vi "m2Triangle.vi"() -> ()   [LabVIEW 2015]
uses:
  Common_RT_ILC/DataTypes/ILCTelemetry.ctl
  Common_RT_ILC/DataTypes/ILCResponses.ctl
  Common_RT_Modbus/DataTypes/ExceptionCodes.ctl
  Common_RT_HPILC/DataTypes/HPResponses.ctl
  Common_RT_HPILC/DataTypes/HPTelemetry.ctl
  Common_RT_HealthAndStatus/RTHealthAndStatus/RTHealthAndStatus.lvclass
  MyHealthAndStatusReadFIFO/MyHealthAndStatusReadFIFO.lvclass
  MyHealthAndStatusWriteFIFO/MyHealthAndStatusWriteFIFO.lvclass
  Common_RT_Modbus/Modbus/Modbus.lvclass
  ModbusPort1ReadFIFO/ModbusPort1ReadFIFO.lvclass
  ModbusPort1WriteFIFO/ModbusPort1WriteFIFO.lvclass
  SoftwareControlledTrigger/SoftwareControlledTrigger.lvclass
  Common_RT_HPILC/HPILCFactory/HPILCFactory.lvclass
  Common_RT_HPILC/DataTypes/HPSettings.ctl
  Common_RT_ILC/DataTypes/ILCSettings.ctl
  SoftwareControlledTrigger/SoftwareControlledTrigger.lvclass/SoftwareControlledTrigger.ctl
  ModbusPort1WriteFIFO/ModbusPort1WriteFIFO.lvclass/ModbusPort1WriteFIFO.ctl
  ModbusPort1ReadFIFO/ModbusPort1ReadFIFO.lvclass/ModbusPort1ReadFIFO.ctl
  MyHealthAndStatusWriteFIFO/MyHealthAndStatusWriteFIFO.lvclass/MyHealthAndStatusWriteFIFO.ctl
  MyHealthAndStatusReadFIFO/MyHealthAndStatusReadFIFO.lvclass/MyHealthAndStatusReadFIFO.ctl
  Common_RT_HealthAndStatus/RTHealthAndStatus/RTHealthAndStatus.lvclass/RTHealthAndStatus.ctl
  Common_RT_ILC/ILC/ILC.lvclass/ILC.ctl
  Common_RT_Modbus/DynamicFrameParser/DynamicFrameParser.lvclass
  Common_RT_HPILC/HPILC/HPILC.lvclass/HPILC.ctl
  <vilib>/FPGAPlugInAG/cRIO-9038/niLvFpga_Open_cRIO-9038.vi
  <vilib>/rvi/interface/common/dynamic/niFpgaDynamicAddResources.vi
  <vilib>/FPGAPlugInAG/Dynamic/niLvFpga_Abort_Dynamic.vi
  <vilib>/FPGAPlugInAG/Dynamic/niLvFpga_Reset_Dynamic.vi
  <vilib>/FPGAPlugInAG/Dynamic/niLvFpga_Run_Dynamic.vi
  <vilib>/Utility/error.llb/Error Cluster From Error Code.vi
  <vilib>/RVI Host/nirviSupport.llb/nirviErrorClusterFromErrorCode.vi
  <vilib>/rvi/errors/niLvFpgaAdjustHostInterfaceError.vi
  <vilib>/FPGAPlugInAG/Dynamic/niLvFpga_Close_Dynamic.vi
  <vilib>/rvi/interface/nirviOpenFPGA/nirviOpenFPGA.xnode
  FPGA Bitfiles/Modbus-4Port.lvbitx
  FPGA/main.vi
  <vilib>/rvi/interface/nirviMethod/nirviMethod.xnode
  <vilib>/rvi/interface/nirviCloseFPGA/nirviCloseFPGA.xnode
  Common_RT_HPILC/HPILC/HPILC.lvclass
  Common_RT_ILC/RTILC.lvlib
  <vilib>/rvi/interface/nirviMethod/StockFPGA_InlinedMethodWaitForSingleIRQ.vi
  <vilib>/FPGAPlugInAG/Dynamic/niLvFpga_WaitOnIrq_Dynamic.vi
  <vilib>/FPGAPlugInAG/Dynamic/niLvFpga_AcknowledgeIrq_Dynamic.vi
  Common_RT_ILC/ILC/ILC.lvclass
  Common_RT_HPILC/RTHPILC.lvlib
  Common_RT_Modbus/RTModbus.lvlib
panel:
  out "minMinEncoder":i32
  out "maxMinEncoder":i32
  out "minMaxEncoder":i32
  out "maxMaxEncoder":i32
  out "Exception on Force and Status":bool
  out "minAvgDelta":dbl
  out "maxAvgDelta":dbl
  out "minMaxDelta":i32
  out "maxMaxDelta":i32
  out "minMinDelta":i32
  out "maxMinDelta":i32
  out "MaxDelta":i32(graph)
  out "MinDelta":i32(graph)
  out "AvgDelta":dbl(graph)
  out "avgDelta":dbl
  out "minDelta":i32
  out "maxDelta":i32
  out "minValue":i32
  out "maxValue":i32
  out "Encoder":i32(graph)
  out "Steps":i32
  in  "Stop":bool
  out "HPTelemetry":T1
  out "HPResponses":T2
  in  "Boolean":bool
  out "ILCResponses":T4
  out "ILCTelemetry":T5
  out "Port 1 Status Bits":u64 format="%016b"
  out "error out":errorcluster
  out "Port 1 Frames Received":i64
  out "Port 1 Bytes Received":i64
  out "Port 1 Frames Transmitted":i64
  out "Port 1 Bytes Transmitted":i64
  # "Port 1 = Modbus"
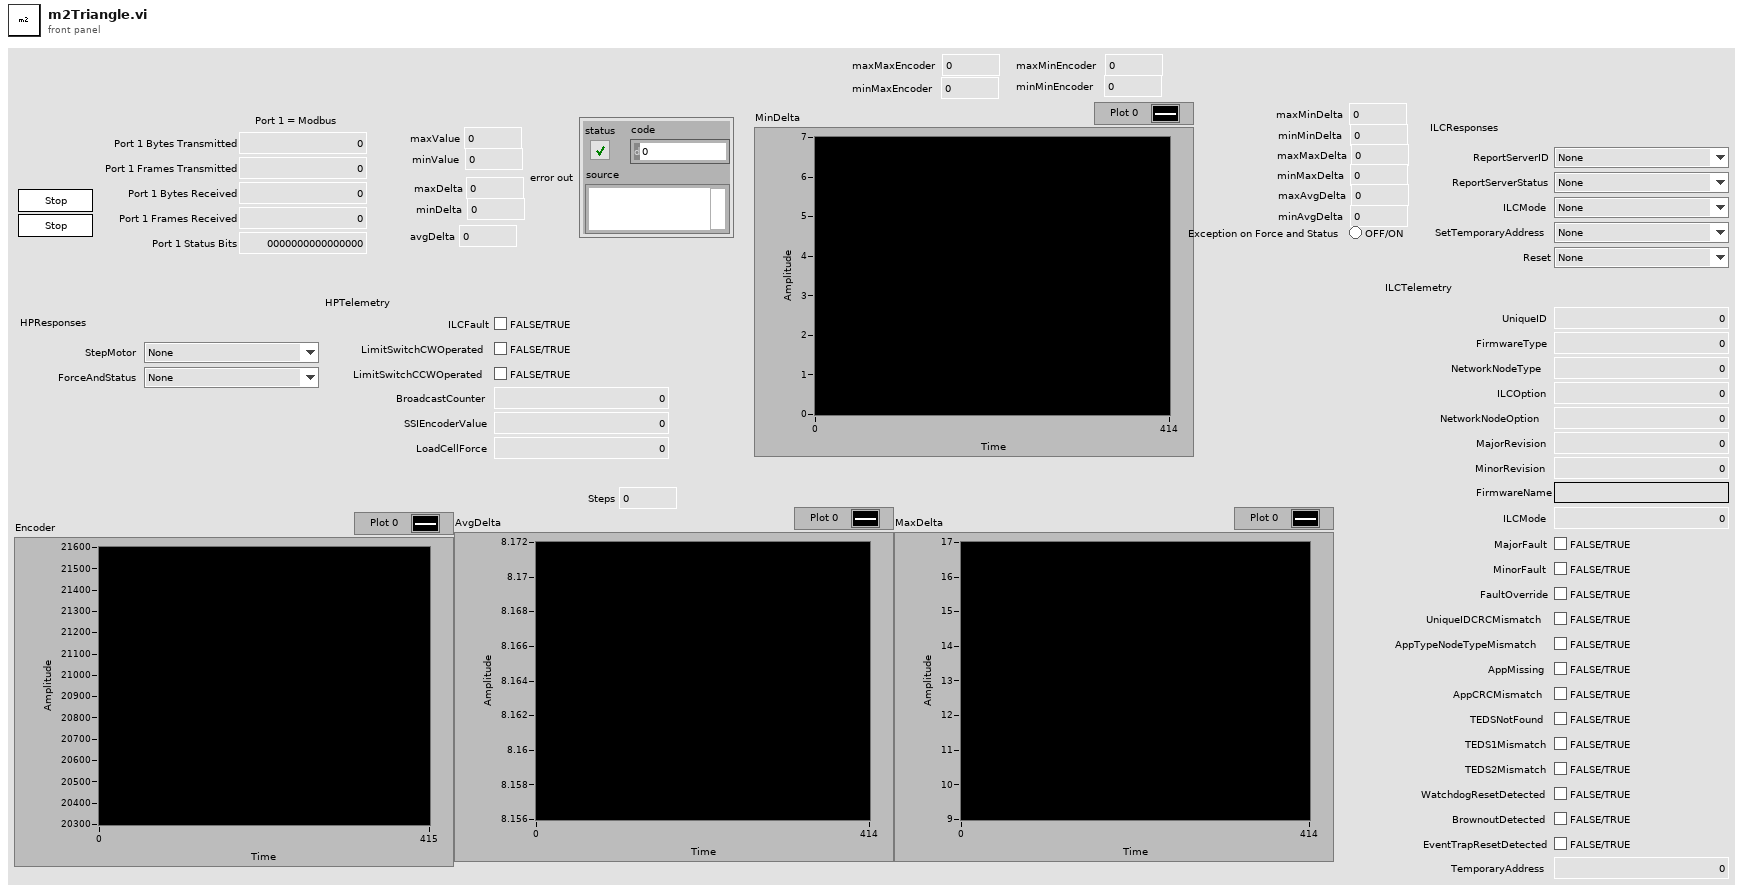
[diagram p1: front panel]
types:
  T1 = typedef "RTHPILC.lvlib/HPTelemetry.ctl" = cluster{"ILCFault":bool, "LimitSwitchCWOperated":bool, "LimitSwitchCCWOperated":bool, "BroadcastCounter":u8, "SSIEncoderValue":i32, "LoadCellForce":sgl}
  T2 = typedef "RTHPILC.lvlib/HPResponses.ctl" = cluster{"StepMotor":T3, "ForceAndStatus":T3}
  T3 = typedef "RTModbus.lvlib/ExceptionCodes.ctl" = enum16{"None", "IllegalFunction", "IllegalDataAddress", "IllegalDataValue", "SlaveDeviceFailure", "Acknowledge", "SlaveDeviceBusy", "NegativeAcknowledge", "MemoryParityError", "GatewayPathUnavailable", "GatewayTargetDeviceFailedToRespond"}
  T4 = typedef "RTILC.lvlib/ILCResponses.ctl" = cluster{"ReportServerID":T3, "ReportServerStatus":T3, "ILCMode":T3, "SetTemporaryAddress":T3, "Reset":T3}
  T5 = typedef "RTILC.lvlib/ILCTelemetry.ctl" = cluster{"UniqueID":u64, "FirmwareType":u8, "NetworkNodeType":u8, "ILCOption":u8, "NetworkNodeOption":u8, "MajorRevision":u8, "MinorRevision":u8, "FirmwareName":string, "ILCMode":u16, "MajorFault":bool, "MinorFault":bool, "FaultOverride":bool, "UniqueIDCRCMismatch":bool, "AppTypeNodeTypeMismatch":bool, "AppMissing":bool, "AppCRCMismatch":bool, "TEDSNotFound":bool, "TEDS1Mismatch":bool, "TEDS2Mismatch":bool, "WatchdogResetDetected":bool, "BrownoutDetected":bool, "EventTrapResetDetected":bool, "TemporaryAddress":u8}
  T6 = typedef "RTHPILC.lvlib/HPSettings.ctl" = cluster{"ILCSettings":T7, "ID":i16, "ReferencePosition":u32}
  T7 = typedef "RTILC.lvlib/ILCSettings.ctl" = cluster{"Subnet":u8, "Address":u8}
  T8 = typedef "RTILC.lvlib/ILCData.ctl" = cluster{"Constants":T9, "Command":T10, "Telemetry":T5, "Responses":T4}
  T9 = typedef "RTILC.lvlib/ILCConstants.ctl" = cluster{"Subnet":u8, "Address":u8}
  T10 = typedef "RTILC.lvlib/ILCCommand.ctl" = cluster{"ILCMode":u16, "TemporaryAddress":u8}
  T11 = typedef "RTModbus.lvlib/Frame.ctl" = cluster{"Data":u8[], "WaitForTrigger":bool, "WaitForRx":u16, "TriggerIRQ":bool}
  T12 = typedef "RTHPILC.lvlib/HPData.ctl" = cluster{"HPConstants":T13, "HPCommand":T14, "HPTelemetry":T1, "HPResponses":T2}
  T13 = typedef "RTHPILC.lvlib/HPConstants.ctl" = cluster{"ID":i16, "ReferencePosition":u32}
  T14 = typedef "RTHPILC.lvlib/HPCommand.ctl" = cluster{"Steps":i8}
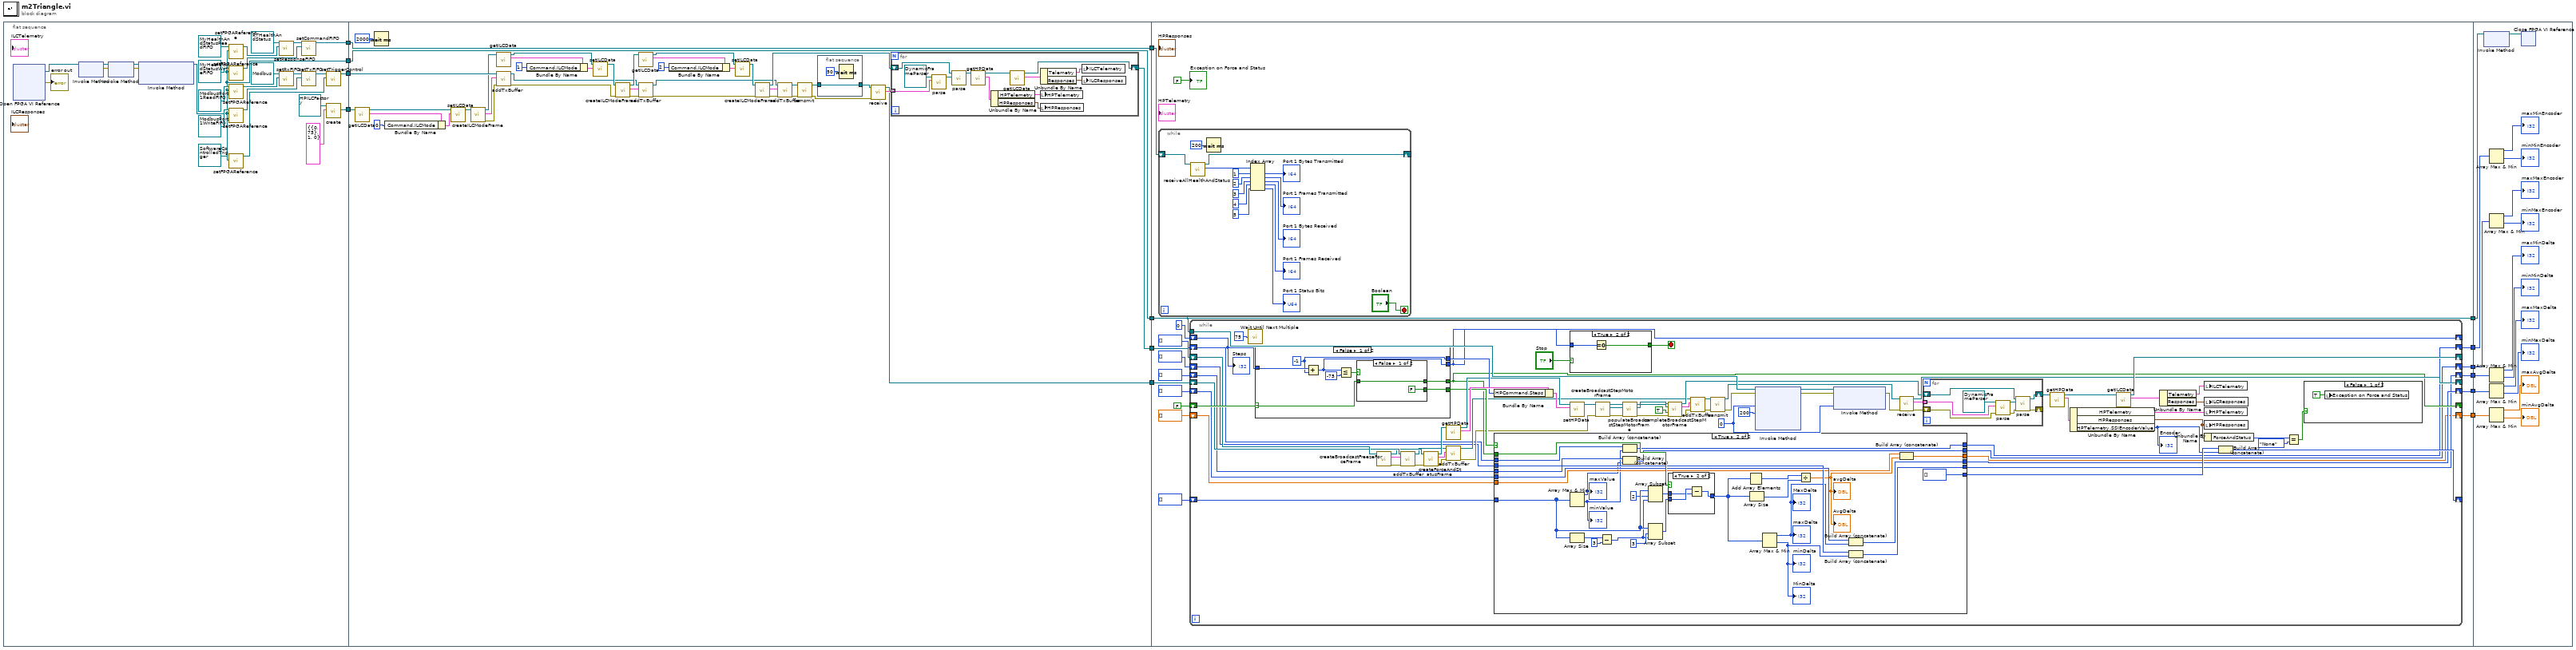
[diagram p0: block diagram]
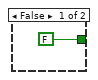
[diagram p3: hidden frame]
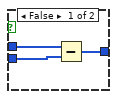
[diagram p5: hidden frame]
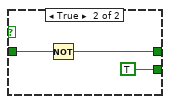
[diagram p6: hidden frame]
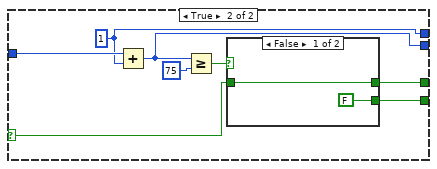
[diagram p7: hidden frame]
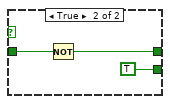
[diagram p8: hidden frame]
diagram:
  n1 = flat-sequence {
    tunnel: [w22] -> w14
    tunnel: [w19] -> w11
    tunnel: [w37] -> w10
    tunnel: [w15] -> w8
    tunnel: w14 -> [w82]
    tunnel: [w82] -> w13
    tunnel: w11 -> [w47]
    tunnel: w10 -> [w80]
    tunnel: [w80] -> w9
    tunnel: w8 -> [w48]
    tunnel: [w57] -> w7
    tunnel: [w56] -> w6
    tunnel: w13 -> [w110]
    tunnel: [w110] -> w12
    tunnel: w9 -> [w115]
    tunnel: w7 -> [w112]
    tunnel: w6 -> [w111]
    tunnel: [w105] -> w5
    tunnel: [w104] -> w4
    tunnel: [w103] -> w3
    tunnel: [w100] -> w2
    tunnel: [w98] -> w1
    tunnel: w12 -> [w298]
    tunnel: w5 -> [w297]
    tunnel: w4 -> [w294]
    tunnel: w3 -> [w291]
    tunnel: w2 -> [w288]
    tunnel: w1 -> [w285]
    frame #0 {
      n2 = xnode "Open FPGA VI Reference"() -> ("FPGA VI Reference Out"=w24:refnum<k20>, "error out"=→"error out":errorcluster)  [unwired: 2 in]
      n3 = xnode "Invoke Method"("FPGA VI Reference In"=w24) -> ("FPGA VI Reference Out"=w41:refnum<k20>, "error out"=w26:errorcluster)  [unwired: 1 in]
      n4 = xnode "Invoke Method"("FPGA VI Reference In"=w41, "error in"=w26) -> ("FPGA VI Reference Out"=w40:refnum<k20>, "error out"=w25:errorcluster)
      n5 = xnode "Invoke Method"("FPGA VI Reference In"=w40, "error in"=w25) -> ("FPGA VI Reference Out"=w22:refnum<k20>)  [unwired: 1 in, 1 out]
      n6 = call "setFPGAReference.vi"("FPGAReference"=w22, "MyHealthAndStatusReadFIFO in"=refnum<class "MyHealthAndStatusReadFIFO.lvclass"> refnum ("MyHealthAndStatusReadFIFO.lvclass")) -> ("MyHealthAndStatusReadFIFO out"=w33:refnum<class "MyHealthAndStatusReadFIFO.lvclass">)  [unwired: 9 in]
      n7 = call "setFPGAReference.vi"("FPGAReference"=w22, "MyHealthAndStatusWriteFIFO in"=refnum<class "MyHealthAndStatusWriteFIFO.lvclass"> refnum ("MyHealthAndStatusWriteFIFO.lvclass")) -> ("MyHealthAndStatusWriteFIFO out"=w31:refnum<class "MyHealthAndStatusWriteFIFO.lvclass">)  [unwired: 9 in]
      n8 = call "setFPGAReference.vi"("FPGAReference"=w22, "ModbusPort1ReadFIFO in"=refnum<class "ModbusPort1ReadFIFO.lvclass"> refnum ("ModbusPort1ReadFIFO.lvclass")) -> ("ModbusPort1ReadFIFO out"=w29:refnum<class "ModbusPort1ReadFIFO.lvclass">)  [unwired: 9 in]
      n9 = call "setFPGAReference.vi"("FPGAReference"=w22, "ModbusPort1WriteFIFO in"=refnum<class "ModbusPort1WriteFIFO.lvclass"> refnum ("ModbusPort1WriteFIFO.lvclass")) -> ("ModbusPort1WriteFIFO out"=w27:refnum<class "ModbusPort1WriteFIFO.lvclass">)  [unwired: 9 in]
      n10 = call "setFPGAReference.vi"("FPGAReference"=w22, "SoftwareControlledTrigger in"=refnum<class "SoftwareControlledTrigger.lvclass"> refnum ("SoftwareControlledTrigger.lvclass")) -> ("SoftwareControlledTrigger out"=w18:refnum<class "SoftwareControlledTrigger.lvclass">)  [unwired: 9 in]
      n11 = call "setResponseFIFO.vi"("ReadU32FIFO"=w33, "RTHealthAndStatus in"=refnum<class "RTHealthAndStatus.lvclass"> refnum ("RTHealthAndStatus.lvlib:RTHealthAndStatus.lvclass")) -> ("RTHealthAndStatus out"=w38:refnum<class "RTHealthAndStatus.lvclass">)  [unwired: 9 in]
      n12 = call-dynamic "setRxFIFO.vi"("ReadU16FIFO"=w29, "Modbus in"=refnum<class "Modbus.lvclass"> refnum ("RTModbus.lvlib:Modbus.lvclass")) -> ("Modbus out"=w35:refnum<class "Modbus.lvclass">)  [unwired: 9 in]
      n13 = call "setCommandFIFO.vi"("WriteU64FIFO"=w31, "RTHealthAndStatus in"=w38) -> ("RTHealthAndStatus out"=w37:refnum<class "RTHealthAndStatus.lvclass">)  [unwired: 9 in]
      n14 = call-dynamic "setTxFIFO.vi"("WriteU16FIFO"=w27, "Modbus in"=w35) -> ("Modbus out"=w20:refnum<class "Modbus.lvclass">)  [unwired: 9 in]
      n15 = call-dynamic "setTriggerControl.vi"("BooleanControl"=w18, "Modbus in"=w20) -> ("Modbus out"=w19:refnum<class "Modbus.lvclass">)  [unwired: 9 in]
      n16 = call "create.vi"("HPSettings"=T6 {"ILCSettings"={"Subnet"=0, "Address"=73}, "ID"=1, "ReferencePosition"=0}, "HardPointActuatorFactory in"=refnum<class "HPILCFactory.lvclass"> refnum ("RTHPILC.lvlib:HPILCFactory.lvclass")) -> ("HardPointActuator"=w15:refnum<class "HPILC.lvclass">)  [unwired: 7 in, 2 out]
    }
    frame #1 {
      n17 = call "getILCData.vi"("ILC in"=w48) -> ("ILCData"=w49:T8, "ILC out"=w53:refnum<class "HPILC.lvclass">)  [unwired: 9 in]
      n18 = Wait (ms)(milliseconds to wait=u32 2000) -> ()  [unwired: 1 out]
      n19 = Bundle By Name(cluster=w49, "Command.ILCMode"=u16 0) -> (w51:T8)
      n20 = call "setILCData.vi"("ILCData"=w51, "ILC in"=w53) -> ("ILC out"=w52:refnum<class "HPILC.lvclass">)  [unwired: 9 in]
      n21 = call "createILCModeFrame.vi"("ILC in"=w52) -> ("error out"=w55:errorcluster, "Frame"=w54:T11, "ILC out"=w46:refnum<class "HPILC.lvclass">)  [unwired: 8 in]
      n22 = call "getILCData.vi"("ILC in"=w46) -> ("ILCData"=w79:T8, "ILC out"=w69:refnum<class "HPILC.lvclass">)  [unwired: 9 in]
      n23 = call-dynamic "addTxBuffer.vi"("error in (no error)"=w55, "Frame"=w54, "Modbus in"=w47) -> ("error out"=w44:errorcluster, "Modbus out"=w45:refnum<class "Modbus.lvclass">)  [unwired: 7 in]
      n24 = Bundle By Name(cluster=w79, "Command.ILCMode"=u16 1) -> (w77:T8)
      n25 = call "setILCData.vi"("ILCData"=w77, "ILC in"=w69) -> ("ILC out"=w70:refnum<class "HPILC.lvclass">)  [unwired: 9 in]
      n26 = call "createILCModeFrame.vi"("error in (no error)"=w44, "ILC in"=w70) -> ("error out"=w66:errorcluster, "Frame"=w68:T11, "ILC out"=w71:refnum<class "HPILC.lvclass">)  [unwired: 7 in]
      n27 = call "getILCData.vi"("ILC in"=w71) -> ("ILCData"=w76:T8, "ILC out"=w73:refnum<class "HPILC.lvclass">)  [unwired: 9 in]
      n28 = call-dynamic "addTxBuffer.vi"("error in (no error)"=w66, "Frame"=w68, "Modbus in"=w45) -> ("error out"=w42:errorcluster, "Modbus out"=w43:refnum<class "Modbus.lvclass">)  [unwired: 7 in]
      n29 = Bundle By Name(cluster=w76, "Command.ILCMode"=u16 2) -> (w74:T8)
      n30 = call "setILCData.vi"("ILCData"=w74, "ILC in"=w73) -> ("ILC out"=w72:refnum<class "HPILC.lvclass">)  [unwired: 9 in]
      n31 = call "createILCModeFrame.vi"("error in (no error)"=w42, "ILC in"=w72) -> ("error out"=w65:errorcluster, "Frame"=w67:T11, "ILC out"=w58:refnum<class "HPILC.lvclass">)  [unwired: 7 in]
      n32 = call-dynamic "addTxBuffer.vi"("error in (no error)"=w65, "Frame"=w67, "Modbus in"=w43) -> ("error out"=w63:errorcluster, "Modbus out"=w64:refnum<class "Modbus.lvclass">)  [unwired: 7 in]
      n33 = call-dynamic "transmit.vi"("error in (no error)"=w63, "Modbus in"=w64) -> ("error out"=w60:errorcluster, "Modbus out"=w62:refnum<class "Modbus.lvclass">)  [unwired: 8 in]
      n34 = flat-sequence {
        tunnel: [w96] -> w61
        tunnel: w62 -> [w96]
        frame #0 {
          n35 = Wait (ms)(milliseconds to wait=u32 50) -> ()  [unwired: 1 out]
        }
      }
      n36 = call-dynamic "receive.vi"("error in (no error)"=w60, "Modbus in"=w61) -> ("Data"=w59:T11[], "Modbus out"=w56:refnum<class "Modbus.lvclass">)  [unwired: 7 in, 1 out]
      n37 = for {
        tunnel: w59 -> [w95] mode=indexing
        shift-right: [w83] -> w57
        shift-left: w58 -> [w92]
        n38 = call "parse.vi"("Frame"=w95, "FrameParser in"=refnum<class "DynamicFrameParser.lvclass"> refnum ("RTModbus.lvlib:DynamicFrameParser.lvclass")) -> ("FrameParser out"=w93:refnum<class "DynamicFrameParser.lvclass">)  [unwired: 8 in, 1 out]
        n39 = call-dynamic "parse.vi"("DynamicFrameParser"=w93, "HPILC in"=w92) -> ("HPILC out"=w84:refnum<class "HPILC.lvclass">)  [unwired: 7 in, 2 out]
        n40 = call "getHPData.vi"("HardPointActuator in"=w84) -> ("HPData"=w85:T12, "HardPointActuator out"=w91:refnum<class "HPILC.lvclass">)  [unwired: 9 in]
        n41 = Unbundle By Name(w85) -> ("HPTelemetry"=w86:T1, "HPResponses"=w87:T2)
        n42 = call "getILCData.vi"("ILC in"=w91) -> ("ILCData"=w88:T8, "ILC out"=w83:refnum<class "HPILC.lvclass">)  [unwired: 9 in]
        n43 = Unbundle By Name(w88) -> ("Telemetry"=w89:T5, "Responses"=w90:T4)
        n44 = local write "HPTelemetry"(w86) -> ()
        n45 = local write "HPResponses"(w87) -> ()
        n46 = local write "ILCTelemetry"(w89) -> ()
        n47 = local write "ILCResponses"(w90) -> ()
      }
    }
    frame #2 {
      n48 = while {
        shift-right: [w280] -> _
        shift-left: w115 -> [w281]
        stop <- "Boolean" stop-if-true
        n49 = call "receiveAllHealthAndStatus.vi"("RTHealthAndStatus in"=w281) -> ("Data"=w275:u32[], "RTHealthAndStatus out"=w280:refnum<class "RTHealthAndStatus.lvclass">)  [unwired: 8 in, 1 out]
        n50 = Wait (ms)(milliseconds to wait=u32 200) -> ()  [unwired: 1 out]
        n51 = Index Array(array=w275, index #1=1 ("index"), index #2=2 ("index"), index #3=3 ("index"), index #4=4 ("index"), index #5=5 ("index")) -> (element #1=→"Port 1 Bytes Transmitted":u32, element #2=→"Port 1 Frames Transmitted":u32, element #3=→"Port 1 Bytes Received":u32, element #4=→"Port 1 Frames Received":u32, element #5=→"Port 1 Status Bits":u32)
      }
      n52 = while {
        shift-right: [w144] -> _
        shift-left: 0 -> [w188]
        shift-right: [w141] -> _
        shift-left: FALSE -> [w189]
        shift-right: [w151] -> _
        shift-left: w112 -> [w185]
        shift-right: [w150] -> _
        shift-left: w111 -> [w168]
        tunnel: w110 -> [w163]
        shift-right: [w145] -> _
        shift-left: i32[] [] -> [w148]
        shift-right: [w139] -> w104
        shift-left: i32[] [] -> [w140]
        shift-right: [w137] -> w105
        shift-left: i32[] [] -> [w138]
        shift-right: [w135] -> w103
        shift-left: dbl[] [] -> [w136]
        shift-right: [w118] -> w100
        shift-left: i32[] [] -> [w119]
        shift-right: [w116] -> w98
        shift-left: i32[] [] -> [w117]
        stop <- w142 stop-if-true
        w164 = 0 ("IRQ Number(s)")
        n53 = call "Wait Until Next Multiple"("Count(mSec)"=u32 75) -> ()  [unwired: 1 out]
        n54 = case shown="False" w189 {
          selector: w189 -> [w246 w259]
          tunnel: w188 -> [w248 w262]
          tunnel: [w245 w258] -> w141
          tunnel: [w244 w257] -> w144
          tunnel: [w243 w256] -> w183
          tunnel: [w242 w255] -> w149
          frame False {
            w243 = -1 ("y")
            n55 = Add(x=w248, y=w243) -> (x+y=w244:i32)
            n56 = Less Or Equal?(x=w244, y=-75) -> (x <= y?=w247:bool)
            n57 = case shown="False" w247 {
              tunnel: w246 -> [w251 w254]
              tunnel: [w251 w253] -> w245
              tunnel: [FALSE TRUE] -> w242
              frame False {
              }
              frame True {
                n58 = Not(x=w254) -> (.not. x?=w253:bool)
              }
            }
          }
          frame True {
            w256 = 1 ("y")
            n59 = Add(x=w262, y=w256) -> (x+y=w257:i32)
            n60 = Greater Or Equal?(x=w257, y=75) -> (x >= y?=w260:bool)
            n61 = case shown="False" w260 {
              tunnel: w259 -> [w264 w266]
              tunnel: [w264 w267] -> w258
              tunnel: [FALSE TRUE] -> w255
              frame False {
              }
              frame True {
                n62 = Not(x=w266) -> (.not. x?=w267:bool)
              }
            }
          }
        }
        n63 = call "createBroadcastFreezeForceFrame.vi"("HardPointActuator in"=w185) -> ("error out"=w186:errorcluster, "Frame"=w187:T11, "HardPointActuator out"=w127:refnum<class "HPILC.lvclass">)  [unwired: 8 in]
        n64 = call-dynamic "addTxBuffer.vi"("error in (no error)"=w186, "Frame"=w187, "Modbus in"=w168) -> ("error out"=w130:errorcluster, "Modbus out"=w124:refnum<class "Modbus.lvclass">)  [unwired: 7 in]
        n65 = call "createForceAndStatusFrame.vi"("error in (no error)"=w130, "HardPointActuator in"=w127) -> ("error out"=w171:errorcluster, "Frame"=w170:T11, "HardPointActuator out"=w126:refnum<class "HPILC.lvclass">)  [unwired: 7 in]
        n66 = call "getHPData.vi"("HardPointActuator in"=w126) -> ("HPData"=w184:T12, "HardPointActuator out"=w181:refnum<class "HPILC.lvclass">)  [unwired: 9 in]
        n67 = call-dynamic "addTxBuffer.vi"("error in (no error)"=w171, "Frame"=w170, "Modbus in"=w124) -> ("error out"=w129:errorcluster, "Modbus out"=w123:refnum<class "Modbus.lvclass">)  [unwired: 7 in]
        n68 = Bundle By Name(cluster=w184, "HPCommand.Steps"=w183) -> (w182:T12)
        n69 = case shown="True" w149 {
          tunnel: w148 -> [w199 w225]
          tunnel: [w199 i32[] []] -> w147
          tunnel: w141 -> [_ w221]
          tunnel: w140 -> [w198 w214]
          tunnel: [w198 w213] -> w139
          tunnel: w138 -> [w197 w212]
          tunnel: [w197 w211] -> w137
          tunnel: w136 -> [w196 w210]
          tunnel: [w196 w209] -> w135
          tunnel: w119 -> [w195 w205]
          tunnel: [w195 w204] -> w118
          tunnel: w117 -> [w194 w202]
          tunnel: [w194 w201] -> w116
          frame False {
          }
          frame True {
            n70 = Array Max & Min(array=w225) -> (max value=w200:i32, min value=w203:i32)  [unwired: 2 out]
            "maxValue" <- w200
            "minValue" <- w203
            n71 = Array Size(array=w225) -> (size(s)=w220:i32)
            n72 = Subtract(x=w220, y=3) -> (x-y=w218:i32)
            n73 = Build Array (concatenate)(w202, w203) -> (w201:i32[])
            n74 = Build Array (concatenate)(w205, w200) -> (w204:i32[])
            n75 = Array Subset(array=w225, index=2, length=w218) -> (w222:i32[])
            n76 = Array Subset(array=w225, index=3, length=w218) -> (w223:i32[])
            n77 = case shown="True" w221 {
              tunnel: w223 -> [w229 w233]
              tunnel: w222 -> [w230 w232]
              tunnel: [w228 w231] -> w217
              frame False {
                n78 = Subtract(x=w230, y=w229) -> (x-y=w228:i32[])
              }
              frame True {
                n79 = Subtract(x=w233, y=w232) -> (x-y=w231:i32[])
              }
            }
            n80 = Add Array Elements(numeric array=w217) -> (sum=w216:i32)
            n81 = Array Size(array=w217) -> (size(s)=w215:i32)
            n82 = Array Max & Min(array=w217) -> (max value=w207:i32, min value=w206:i32)  [unwired: 2 out]
            "maxDelta" <- w207
            "minDelta" <- w206
            "MaxDelta" <- w207
            "MinDelta" <- w206
            n83 = Divide(x=w216, y=w215) -> (x/y=w208:dbl)
            "avgDelta" <- w208
            "AvgDelta" <- w208
            n84 = Build Array (concatenate)(w214, w207) -> (w213:i32[])
            n85 = Build Array (concatenate)(w212, w206) -> (w211:i32[])
            n86 = Build Array (concatenate)(w210, w208) -> (w209:dbl[])
          }
        }
        n87 = case shown="True" "Stop" {
          tunnel: w144 -> [_ w193]
          tunnel: [FALSE w192] -> w142
          frame False {
          }
          frame True {
            n88 = Equal To 0?(x=w193) -> (x = 0?=w192:bool)
          }
        }
        n89 = call "setHPData.vi"("HPData"=w182, "HardPointActuator in"=w181) -> ("HardPointActuator out"=w180:refnum<class "HPILC.lvclass">)  [unwired: 9 in]
        n90 = call "createBroadcastStepMotorFrame.vi"("error in (no error)"=w129, "HardPointActuator in"=w180) -> ("error out"=w177:errorcluster, "FixedFrameBuilder"=w178:refnum<class "FixedFrameBuilder.lvclass">, "HardPointActuator out"=w179:refnum<class "HPILC.lvclass">)  [unwired: 7 in]
        n91 = call "populateBroadcastStepMotorFrame.vi"("error in (no error)"=w177, "FixedFrameBuilder in"=w178, "HardPointActuator in"=w179) -> ("error out"=w176:errorcluster, "FixedFrameBuilder out"=w175:refnum<class "FixedFrameBuilder.lvclass">, "HardPointActuator out"=w174:refnum<class "HPILC.lvclass">)  [unwired: 6 in]
        n92 = call "completeBroadcastStepMotorFrame.vi"("HardPointActuator in"=w174, "FixedFrameBuilder"=w175, "TriggerIRQ"=TRUE, "error in (no error)"=w176) -> ("HardPointActuator out"=w125:refnum<class "HPILC.lvclass">, "Frame"=w173:T11, "error out"=w172:errorcluster)  [unwired: 9 in]
        n93 = call-dynamic "addTxBuffer.vi"("error in (no error)"=w172, "Frame"=w173, "Modbus in"=w123) -> ("error out"=w128:errorcluster, "Modbus out"=w122:refnum<class "Modbus.lvclass">)  [unwired: 7 in]
        n94 = call-dynamic "transmit.vi"("error in (no error)"=w128, "Modbus in"=w122) -> ("error out"=w167:errorcluster, "Modbus out"=w161:refnum<class "Modbus.lvclass">)  [unwired: 8 in]
        n95 = xnode "Invoke Method"("FPGA VI Reference In"=w163, "error in"=w167, "IRQ Number(s)"=w164, "Timeout (ms)"=200) -> ("FPGA VI Reference Out"=w162:refnum<k20>, "error out"=w165:errorcluster)  [unwired: 2 out]
        n96 = xnode "Invoke Method"("FPGA VI Reference In"=w162, "error in"=w165, "IRQ Number(s)"=w164) -> ("error out"=w160:errorcluster)  [unwired: 1 out]
        n97 = call-dynamic "receive.vi"("error in (no error)"=w160, "Modbus in"=w161) -> ("error out"=w159:errorcluster, "Data"=w120:T11[], "Modbus out"=w150:refnum<class "Modbus.lvclass">)  [unwired: 7 in]
        n98 = for {
          tunnel: w120 -> [w238] mode=indexing
          shift-right: [w236] -> w156
          shift-left: w125 -> [w237]
          shift-right: [w234] -> _
          shift-left: w159 -> [w235]
          n99 = call "parse.vi"("error in (no error)"=w235, "Frame"=w238, "FrameParser in"=refnum<class "DynamicFrameParser.lvclass"> refnum ("RTModbus.lvlib:DynamicFrameParser.lvclass")) -> ("error out"=w239:errorcluster, "FrameParser out"=w240:refnum<class "DynamicFrameParser.lvclass">)  [unwired: 7 in]
          n100 = call-dynamic "parse.vi"("error in (no error)"=w239, "DynamicFrameParser"=w240, "HPILC in"=w237) -> ("error out"=w234:errorcluster, "HPILC out"=w236:refnum<class "HPILC.lvclass">)  [unwired: 6 in, 1 out]
        }
        n101 = call "getHPData.vi"("HardPointActuator in"=w156) -> ("HPData"=w158:T12, "HardPointActuator out"=w152:refnum<class "HPILC.lvclass">)  [unwired: 9 in]
        n102 = Unbundle By Name(w158) -> ("HPTelemetry"=w157:T1, "HPResponses"=w134:T2, "HPTelemetry.SSIEncoderValue"=w146:i32)
        "Encoder" <- w146
        n103 = call "getILCData.vi"("ILC in"=w152) -> ("ILCData"=w155:T8, "ILC out"=w151:refnum<class "HPILC.lvclass">)  [unwired: 9 in]
        n104 = Unbundle By Name(w155) -> ("Telemetry"=w154:T5, "Responses"=w153:T4)
        n105 = local write "ILCTelemetry"(w154) -> ()
        n106 = local write "ILCResponses"(w153) -> ()
        n107 = local write "HPTelemetry"(w157) -> ()
        n108 = local write "HPResponses"(w134) -> ()
        n109 = Unbundle By Name(w134) -> ("ForceAndStatus"=w133:T3)
        n110 = Build Array (concatenate)(w147, w146) -> (w145:i32[])
        n111 = Equal?(x=w133, y=ExceptionCodes."None") -> (x = y?=w131:bool)
        n112 = case shown="False" w131 {
          frame False {
            n113 = local write "Exception on Force and Status"(TRUE ("Boolean 2")) -> ()
          }
          frame True {
          }
        }
        "Steps" <- w188
      }
      "Exception on Force and Status" <- FALSE
    }
    frame #3 {
      n114 = xnode "Invoke Method"("FPGA VI Reference In"=w298) -> ("FPGA VI Reference Out"=w299:refnum<k20>)  [unwired: 1 in, 1 out]
      n115 = Array Max & Min(array=w285) -> (max value=→"maxMinEncoder":i32, min value=→"minMinEncoder":i32)  [unwired: 2 out]
      n116 = Array Max & Min(array=w288) -> (max value=→"maxMaxEncoder":i32, min value=→"minMaxEncoder":i32)  [unwired: 2 out]
      n117 = Array Max & Min(array=w297) -> (max value=→"maxMinDelta":i32, min value=→"minMinDelta":i32)  [unwired: 2 out]
      n118 = Array Max & Min(array=w294) -> (max value=→"maxMaxDelta":i32, min value=→"minMaxDelta":i32)  [unwired: 2 out]
      n119 = Array Max & Min(array=w291) -> (max value=→"maxAvgDelta":dbl, min value=→"minAvgDelta":dbl)  [unwired: 2 out]
      n120 = xnode "Close FPGA VI Reference"("FPGA VI Reference In"=w299) -> ()  [unwired: 1 in, 1 out]
    }
  }
